vi "Start.vi"(8 "error in (no error)":errorcluster, 10 "Model in":refnum<class "Model.lvclass">, 11 "Standby State in":refnum<class "Standby State.lvclass">) -> (0 "error out":errorcluster, 2 "Model out":refnum<class "Model.lvclass">, 3 "Standby State out":refnum<class "Standby State.lvclass">)   [LabVIEW 2016, in "Standby State.lvclass"]
uses:
  Standby State.lvclass
  Model/Model/Model.lvclass
  Typedefs/StateTypes.ctl
  Typedefs/M1M3SupportEUI_TypeDefs.lvlib
  Model/Boot Loader/Boot Loader.lvclass
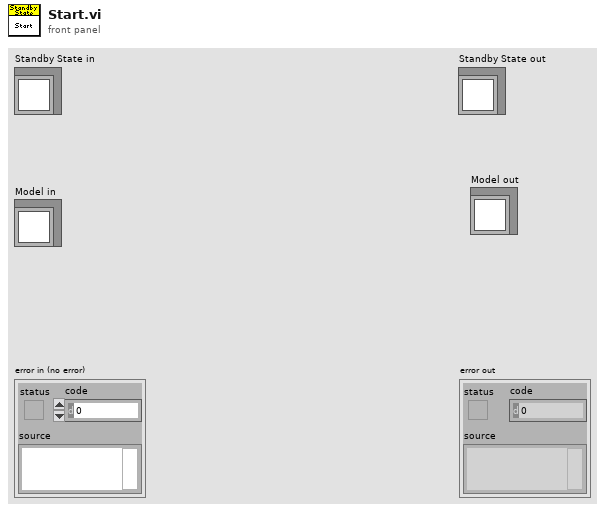
[diagram p1: front panel]
types:
  T1 = typedef "M1M3SupportEUI_TypeDefs.lvlib/StateTypes.ctl" = enum16{"Offline State", "Fault State", "Standby State", "Disabled State", "Enabled State", "Wait For User Input State", "Test Actuator State"}
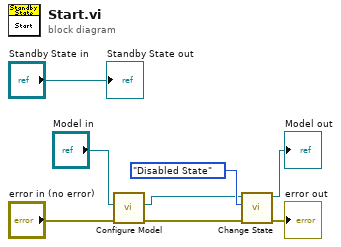
[diagram p0: block diagram]
diagram:
  n1 = call "Configure Model.vi"("error in (no error)"="error in (no error)", "Model in"="Model in") -> ("error out"=w1:errorcluster, "Model out"=w2:refnum<class "Model.lvclass">)  [unwired: 7 in, 1 out]
  n2 = call "Change State.vi"("error in (no error)"=w1, "State Types"=StateTypes."Disabled State" ("State:"), "Model in"=w2) -> ("error out"=→"error out":errorcluster, "Model out"=→"Model out":refnum<class "Model.lvclass">)  [unwired: 7 in]
  "Standby State out" <- "Standby State in"
